vi "Read_Code.vi"(0 "ADC":T1, 1 "Device_no":u16=9 min=1 max=100, 2 "Repeat":i32=2 min=1 max=100, 5 "Port_No":u16=1444, 7 "Core_No":u16=1, 9 "ADC_Controls":T2={"ACQPS"=8, "Ref_Sel(Int/Ext)"=1, "Break_PT"=0, "Ref-Mode_Sel"=0}, 11 "error in":errorcluster) -> (6 "AvgCode":dbl=2.921046198973356, 15 "error out":errorcluster)   [LabVIEW 2019]
uses:
  ADC_CTRL.ctl
  <userlib>/_TI-LA/Reusable/CCS/APIs/Data/Polymorphics/Read Data From Address - U16 Array.vi
  <userlib>/_TI-LA/Reusable/CCS/APIs/CCS.lvlib
panel:
  out "Tot-Error":u32
  out "min value":u32
  out "max value":u32
  out "Voltage":dbl
  out "ADC_No":u16
  out "Waveform Graph":u32[](graph)
  out "Read Data[]":u32[](array[numeric]) format="%#.0f"
  # "Int-0/Ext-1_Sel"
  # "1P65-0/2P5-1_Mode_Sel"
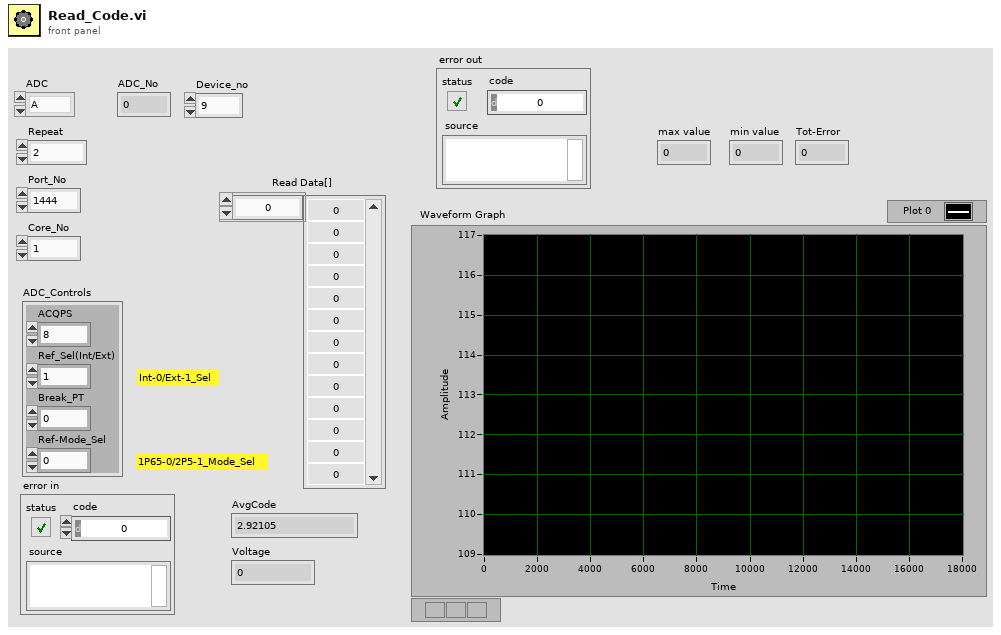
[diagram p1: front panel]
types:
  T1 = typedef "ADC_CTRL.ctl" = enum16{"A", "B", "C"}
  T2 = cluster{"ACQPS":u16, "Ref_Sel(Int/Ext)":u16, "Break_PT":u16, "Ref-Mode_Sel":u16}
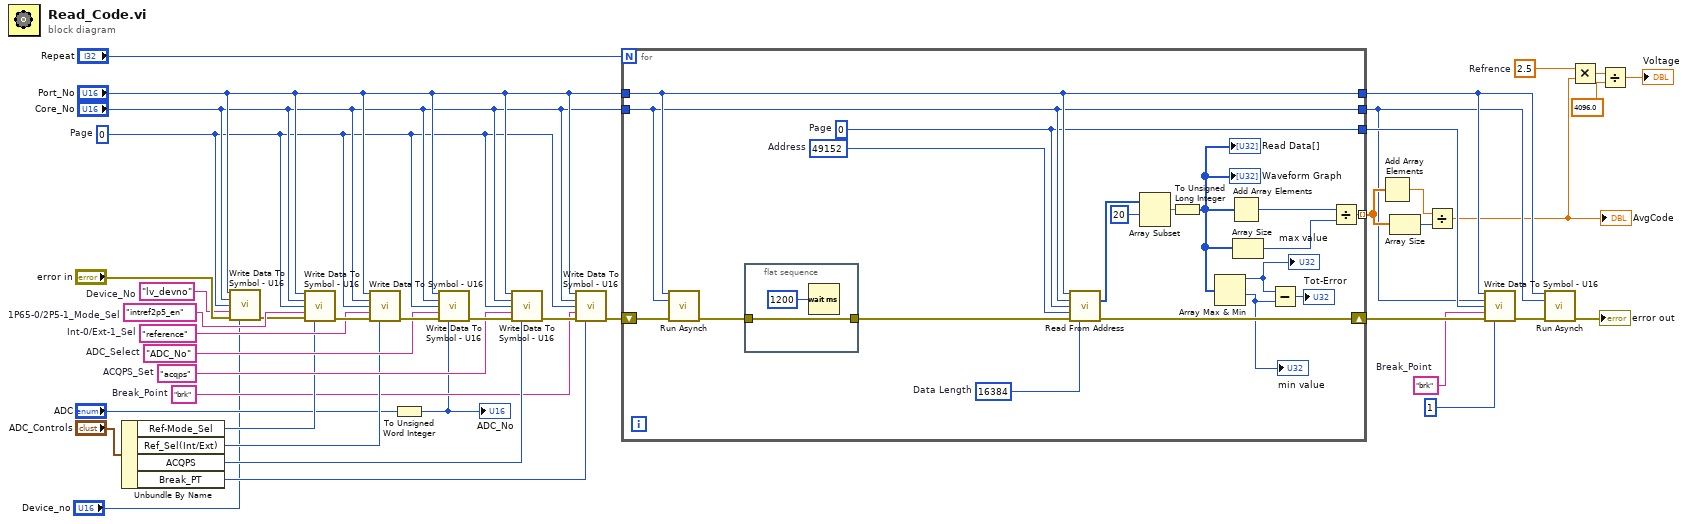
[diagram p0: block diagram]
diagram:
  w5 = "lv_devno"  # Device_No
  w11 = 2.5  # Refrence
  w22 = "brk"  # Break_Point
  w2 = 0  # Page
  w38 = "intref2p5_en"  # 1P65-0/2P5-1_Mode_Sel
  w35 = "acqps"  # ACQPS_Set
  w29 = "brk"  # Break_Point
  w37 = "reference"  # Int-0/Ext-1_Sel
  w36 = "ADC_No"  # ADC_Select
  n1 = Unbundle By Name("ADC_Controls") -> ("Ref-Mode_Sel"=w34:u16, "Ref_Sel(Int/Ext)"=w33:u16, "ACQPS"=w32:u16, "Break_PT"=w21:u16)
  n2 = call <userlib>:"Write Data To Symbol - U16.vi"("Port Number"="Port_No", "Core Number"="Core_No", "Page"=w2, "Symbol Name"=w5, "error in"="error in", "Write Data"="Device_no") -> ("error out"=w7:errorcluster)  [unwired: 7 in, 2 out]
  n3 = call <userlib>:"Write Data To Symbol - U16.vi"("Port Number"="Port_No", "Core Number"="Core_No", "Page"=w2, "Symbol Name"=w38, "error in"=w7, "Write Data"=w34) -> ("error out"=w40:errorcluster)  [unwired: 7 in, 2 out]
  n4 = call <userlib>:"Write Data To Symbol - U16.vi"("Port Number"="Port_No", "Core Number"="Core_No", "Page"=w2, "Symbol Name"=w37, "error in"=w40, "Write Data"=w33) -> ("error out"=w39:errorcluster)  [unwired: 7 in, 2 out]
  n5 = To Unsigned Word Integer(number="ADC") -> (unsigned 16bit integer=w13:u16)
  "ADC_No" <- w13
  n6 = call <userlib>:"Write Data To Symbol - U16.vi"("Port Number"="Port_No", "Core Number"="Core_No", "Page"=w2, "Symbol Name"=w36, "error in"=w39, "Write Data"=w13) -> ("error out"=w41:errorcluster)  [unwired: 7 in, 2 out]
  n7 = call <userlib>:"Write Data To Symbol - U16.vi"("Port Number"="Port_No", "Core Number"="Core_No", "Page"=w2, "Symbol Name"=w35, "error in"=w41, "Write Data"=w32) -> ("error out"=w24:errorcluster)  [unwired: 7 in, 2 out]
  n8 = call <userlib>:"Write Data To Symbol - U16.vi"("Port Number"="Port_No", "Core Number"="Core_No", "Page"=w2, "Symbol Name"=w22, "error in"=w24, "Write Data"=w21) -> ("error out"=w23:errorcluster)  [unwired: 7 in, 2 out]
  n9 = for {
    N: "Repeat" -> [_]
    tunnel: [w54] -> w28 mode=indexing
    tunnel: "Port_No" -> [w49]
    tunnel: "Core_No" -> [w48]
    shift-right: [w52] -> w30
    shift-left: w23 -> [w51]
    tunnel: [w49] -> w19
    tunnel: [w48] -> w18
    tunnel: [w47] -> w25
    w58 = u32 16384  # Data Length
    w59 = u32 49152  # Address
    w47 = 0  # Page
    n10 = call <userlib>:"Run Asynch.vi"("Port Number"=w49, "Core Number"=w48, "error in"=w51) -> ("error out"=w60:errorcluster)  [unwired: 10 in, 2 out]
    n11 = flat-sequence {
      tunnel: w60 -> [w61]
      tunnel: [w61] -> w46
      frame #0 {
        n12 = Wait (ms)(milliseconds to wait=u32 1200) -> ()  [unwired: 1 out]
      }
    }
    n13 = call-poly <userlib>:"Read From Address.vi"("Port Number"=w49, "Core Number"=w48, "Page"=w47, "Address"=w59, "error in"=w46, "Data Length"=w58) -> ("Read Data[]"=w55:u16[], "error out"=w52:errorcluster)  [unwired: 6 in, 2 out]
    n14 = Array Subset(array=w55, index=20) -> (w53:u16[])  [unwired: 1 in]
    n15 = To Unsigned Long Integer(number=w53) -> (unsigned 32bit integer=w45:u32[])
    "Waveform Graph" <- w45
    "Read Data[]" <- w45
    n16 = Array Max & Min(array=w45) -> (max value=w44:u32, min value=w43:u32)  [unwired: 2 out]
    "max value" <- w44
    "min value" <- w43
    n17 = Add Array Elements(numeric array=w45) -> (sum=w57:u32)
    n18 = Array Size(array=w45) -> (size(s)=w50:i32)
    n19 = Subtract(x=w44, y=w43) -> (x-y=→"Tot-Error":u32)
    n20 = Divide(x=w57, y=w50) -> (x/y=w54:dbl)
  }
  n21 = Add Array Elements(numeric array=w28) -> (sum=w26:dbl)
  n22 = Array Size(array=w28) -> (size(s)=w27:i32)
  n23 = Divide(x=w26, y=w27) -> (x/y=w12:dbl)
  "AvgCode" <- w12
  n24 = call <userlib>:"Write Data To Symbol - U16.vi"("Port Number"=w19, "Core Number"=w18, "Page"=w25, "Symbol Name"=w29, "error in"=w30, "Write Data"=u16 1) -> ("error out"=w20:errorcluster)  [unwired: 7 in, 2 out]
  n25 = call <userlib>:"Run Asynch.vi"("Port Number"=w19, "Core Number"=w18, "error in"=w20) -> ("error out"=→"error out":errorcluster)  [unwired: 10 in, 2 out]
  n26 = Multiply(x=w11, y=w12) -> (x*y=w10:dbl)
  n27 = Divide(x=w10, y=4096.0) -> (x/y=→"Voltage":dbl)
